vi "Write Master Timing Module.vi"(8 "error in":errorcluster, 10 "Master Timing Module":string, 11 "Standard Engine Repo Data in":refnum<class "Standard Engine Configuration.lvclass">) -> (0 "error out":errorcluster, 3 "Standard Engine Repo Data out":refnum<class "Standard Engine Configuration.lvclass">)   [LabVIEW 2013, in "Standard Engine Configuration.lvclass"]
doc: "Specify which module (by its identifier) will be used as the engine timing source if the Timing Source Type property is set to \"Use Module Timing Source\"."
uses:
  Standard Engine Configuration.lvclass
  Standard Engine Configuration.lvclass/Standard Engine Configuration.ctl
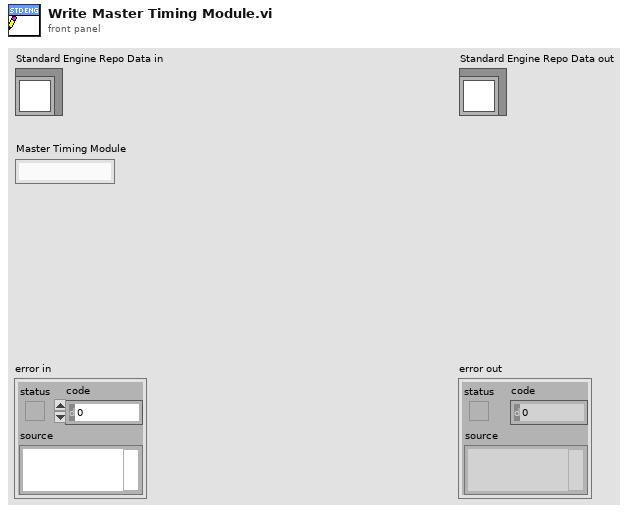
[diagram p1: front panel]
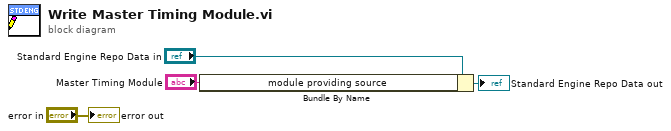
[diagram p0: block diagram]
diagram:
  n1 = Bundle By Name(cluster="Standard Engine Repo Data in", "module providing source"="Master Timing Module") -> (→"Standard Engine Repo Data out":refnum<class "Standard Engine Configuration.lvclass">)
  "error out" <- "error in"
